vi "Create Icon.vi"(8 "error in":errorcluster, 9 "Icon Colors":T1={"Text Color"=0, "Background Color"=16448250, "Border Color"=16746744}, 10 "Icon Text":T2={"Line 1 text"="Example", "Line 2 text"="Test", "Line 3 text"="Bottom", "Line 4 text"=""}) -> (0 "error out":errorcluster, 2 "Picture":picture)   [LabVIEW 2014, in "LabVIEW Icon API.lvlib"]
doc: "Uses a modified example from the LabVIEW Icon API to generate an Icon with the specifed text and coloring."
uses:
  <vilib>/LabVIEW Icon API/LabVIEW Icon API.lvlib
  <vilib>/LabVIEW Icon API/API_Text.ctl
  Icon Editor/Icon Editor.llb/Icon Colors.ctl
  <vilib>/LabVIEW Icon API/lv_icon/Classes/Icon/Icon.lvclass
  <vilib>/LabVIEW Icon API/API_Text Colors.ctl
  <vilib>/LabVIEW Icon API/API_Test Settings.ctl
  <vilib>/LabVIEW Icon API/lv_icon/Controls/Alignment.ctl
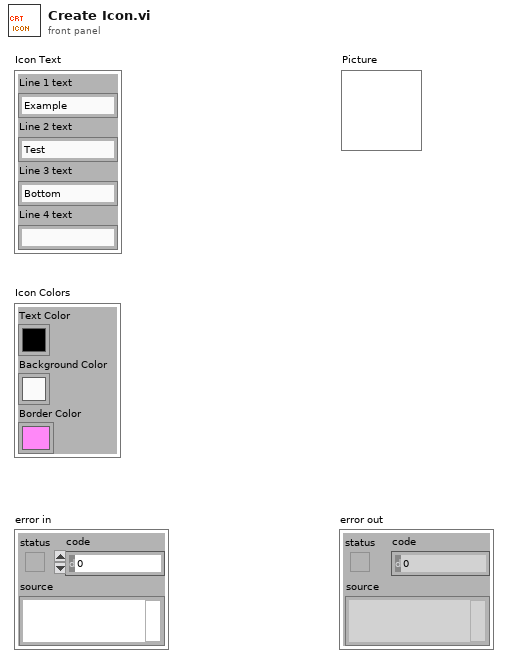
[diagram p1: front panel]
types:
  T1 = typedef "Icon Colors.ctl" = cluster{"Text Color":u32, "Background Color":u32, "Border Color":u32}
  T2 = typedef "LabVIEW Icon API.lvlib/API_Text.ctl" = cluster{"Line 1 text":string, "Line 2 text":string, "Line 3 text":string, "Line 4 text":string}
  T3 = typedef "LabVIEW Icon API.lvlib/API_Test Settings.ctl" = cluster{"Font":string, "Alignment":T4, "Size":u8, "Center text":bool, "Capitalize text":bool, "Text color":T5}
  T4 = typedef "Alignment.ctl" = u16
  T5 = typedef "LabVIEW Icon API.lvlib/API_Text Colors.ctl" = cluster{"Line 1 color":u32, "Line 2 color":u32, "Line 3 color":u32, "Line 4 color":u32}
  T6 = typedef "imagedata.ctl" = cluster{"image type":i32, "image depth":i32, "image":u8[], "mask":u8[], "colors":u32[], "Rectangle":cluster{"left":i16, "top":i16, "right":i16, "bottom":i16}}
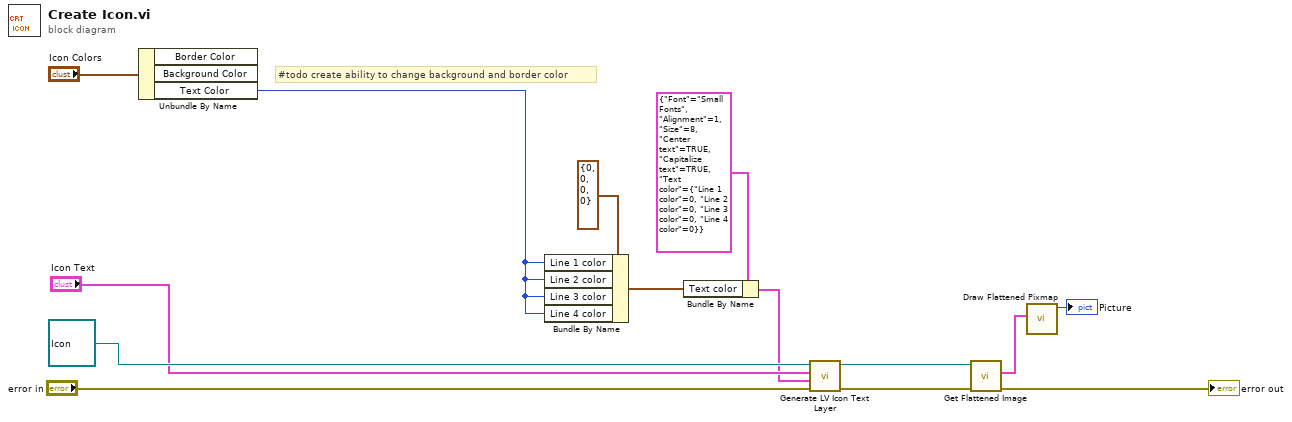
[diagram p0: block diagram]
diagram:
  # "#todo create ability to change background and border color"
  n1 = Unbundle By Name("Icon Colors") -> ("Text Color"=w3:u32)  [unwired: 2 out]
  n2 = Bundle By Name(cluster=T5 {"Line 1 color"=0, "Line 2 color"=0, "Line 3 color"=0, "Line 4 color"=0} ("Text color"), "Line 1 color"=w3, "Line 2 color"=w3, "Line 3 color"=w3, "Line 4 color"=w3) -> (w5:T5)
  n3 = Bundle By Name(cluster=T3 {"Font"="Small Fonts", "Alignment"=1, "Size"=8, "Center text"=TRUE, "Capitalize text"=TRUE, "Text color"={"Line 1 color"=0, "Line 2 color"=0, "Line 3 color"=0, "Line 4 color"=0}} ("Text settings"), "Text color"=w5) -> (w4:T3)
  n4 = call <vilib>:"Generate LV Icon Text Layer.vi"("error in (no error)"="error in", "Text settings"=w4, "Text"="Icon Text", "Icon in"=refnum<class "Icon.lvclass"> refnum ("Icon.lvclass in")) -> ("error out"=w1:errorcluster, "Icon out"=w2:refnum<class "Icon.lvclass">)  [unwired: 6 in]
  n5 = call <vilib>:"Get Flattened Image.vi"("error in (no error)"=w1, "lv_icon.lvlib:Icon.lvclass in"=w2) -> ("error out"=→"error out":errorcluster, "Color Image"=w12:T6)  [unwired: 6 in, 2 out]
  n6 = call <vilib>:"Draw Flattened Pixmap.vi"("image data"=w12) -> ("new picture"=→"Picture":picture)  [unwired: 8 in]
